vi "clone.vi"(0 "reference":refnum<class "StateNode.lvclass">, 5 "error in (no error)":errorcluster) -> (14 "reference out":refnum<class "StateNode.lvclass">, 15 "clonedInterfaceNode":refnum<class "AbstractNode.lvclass">, 19 "error out":errorcluster)   [LabVIEW 2014, in "StateNode.lvclass"]
doc: "public Object clone()"
uses:
  <resource>/Framework/Providers/Open_GDS/UML/StateNode_class/StateNode.lvclass
  <resource>/Framework/Providers/Open_GDS/UML/AbstractNode_class/AbstractNode.lvclass
  <resource>/Framework/Providers/Open_GDS/UML/MultiLineString_class/MultiLineString.lvclass
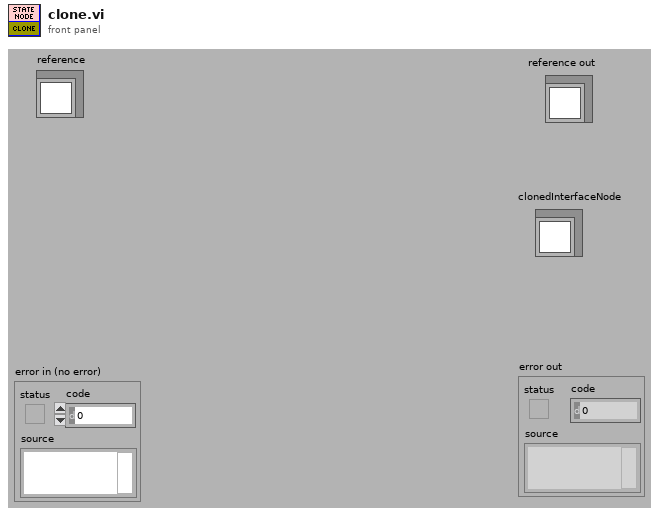
[diagram p1: front panel]
types:
  T1 = typedef "StateNode.lvclass/ObjectAttributes.ctl" = cluster{"Base class":T2, "state":refnum<class "MultiLineString.lvclass">, "action":refnum<class "MultiLineString.lvclass">, "DEFAULT_WIDTH":i32, "DEFAULT_HEIGHT":i32}
  T2 = typedef "RectangularNode.lvclass/ObjectAttributes.ctl" = cluster{"Base class":T3, "bounds":T4}
  T3 = typedef "AbstractNode.lvclass/ObjectAttributes.ctl" = cluster{"parent":refnum<class "AbstractNode.lvclass">, "children":refnum<class "AbstractNode.lvclass">[], "Hidden":bool}
  T4 = typedef "Rectangle Rectangle2D.ctl" = cluster{"x":dbl, "y":dbl, "width":dbl, "height":dbl}
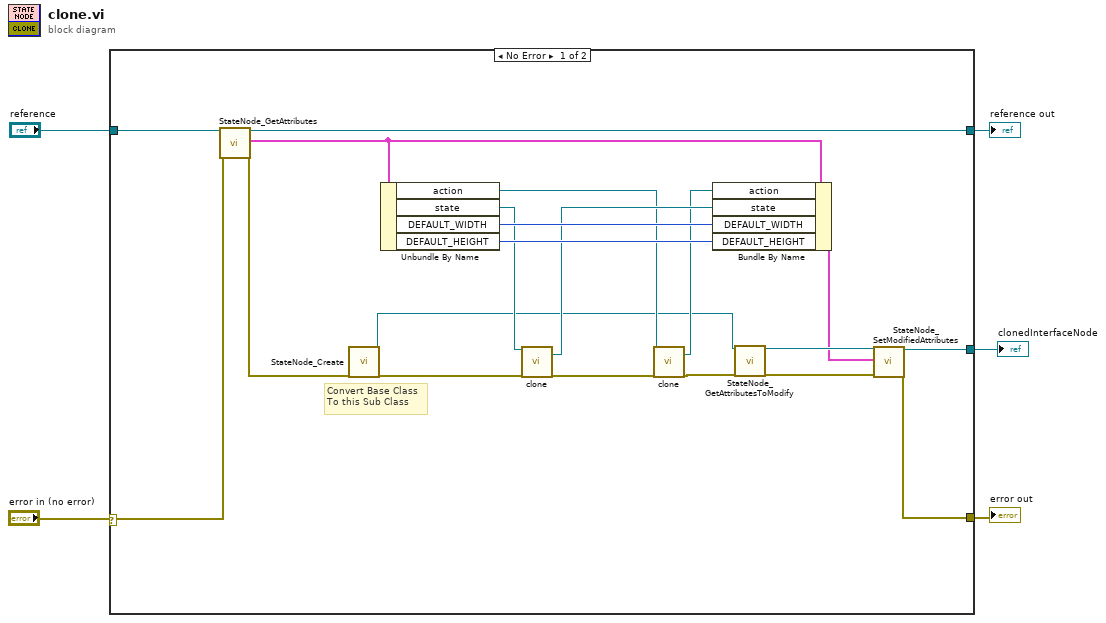
[diagram p0: block diagram]
diagram:
  n1 = case shown="No Error" "error in (no error)" {
    selector: "error in (no error)" -> [w23 w26]
    tunnel: "reference" -> [w25 w27]
    tunnel: [w24 w26] -> w4
    tunnel: [w7 w27] -> w3
    tunnel: [w22 _] -> w1
    frame No Error {
      # "Convert Base Class\nTo this Sub Class"
      n2 = call <resource>:"StateNode_GetAttributes.vi"("reference in"=w25, "error in (no error)"=w23) -> ("reference out"=w7:refnum<class "StateNode.lvclass">, "Attributes"=w8:T1, "error out"=w6:errorcluster)  [unwired: 15 out]
      n3 = call <resource>:"StateNode_Create.vi"("error in (no error)"=w6) -> ("reference out"=w9:refnum<class "StateNode.lvclass">, "error out"=w16:errorcluster)  [unwired: 16 in, 1 out]
      n4 = Unbundle By Name(w8) -> ("action"=w12:refnum<class "MultiLineString.lvclass">, "state"=w15:refnum<class "MultiLineString.lvclass">, "DEFAULT_WIDTH"=w18:i32, "DEFAULT_HEIGHT"=w17:i32)
      n5 = call-dynamic "clone.vi"("reference"=w15, "error in (no error)"=w16) -> ("clonedMultiLineString"=w14:refnum<class "MultiLineString.lvclass">, "error out"=w13:errorcluster)  [unwired: 15 in, 1 out]
      n6 = call-dynamic "clone.vi"("reference"=w12, "error in (no error)"=w13) -> ("clonedMultiLineString"=w11:refnum<class "MultiLineString.lvclass">, "error out"=w10:errorcluster)  [unwired: 15 in, 1 out]
      n7 = Bundle By Name(cluster=w8, "action"=w11, "state"=w14, "DEFAULT_WIDTH"=w18, "DEFAULT_HEIGHT"=w17) -> (w19:T1)
      n8 = call <resource>:"StateNode_GetAttributesToModify.vi"("reference in"=w9, "error in (no error)"=w10) -> ("reference out"=w21:refnum<class "StateNode.lvclass">, "error out"=w20:errorcluster)  [unwired: 1 in, 15 out]
      n9 = call <resource>:"StateNode_SetModifiedAttributes.vi"("reference in"=w21, "Attributes"=w19, "error in (no error)"=w20) -> ("reference out"=w22:refnum<class "StateNode.lvclass">, "error out"=w24:errorcluster)  [unwired: 3 in, 12 out]
    }
    frame Error {
    }
  }
  "reference out" <- w3
  "error out" <- w4
  "clonedInterfaceNode" <- w1
